vi "Cart Type Check.vi"(11 "Main References":T1) -> (1 "Cart type":string, 3 "Same Cart Type?":bool)   [LabVIEW 2020]
uses:
  Main Refs.ctl
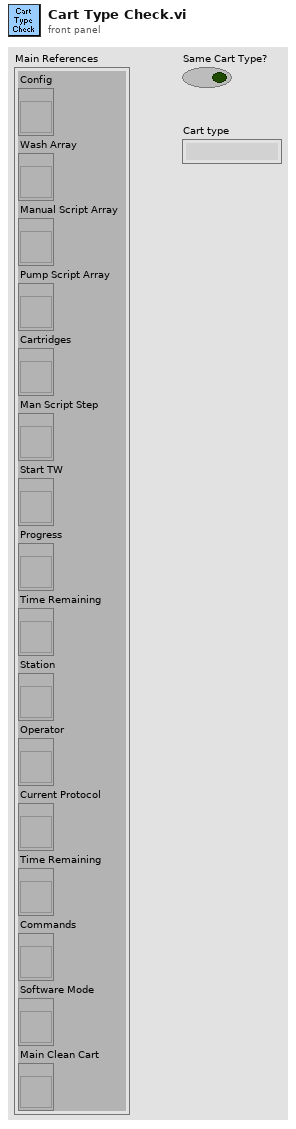
[diagram p1: front panel]
types:
  T1 = typedef "Main Refs.ctl" = cluster{"Config":refnum<vi>, "Wash Array":refnum<vi>, "Manual Script Array":refnum<vi>, "Pump Script Array":refnum<vi>, "Cartridges":refnum<vi>, "Man Script Step":refnum<vi>, "Start TW":refnum<vi>, "Progress":refnum<vi>, "Time Remaining":refnum<vi>, "Station":refnum<vi>, "Operator":refnum<vi>, "Current Protocol":refnum<vi>, "Time Remaining":refnum<vi>, "Commands":refnum<vi>, "Software Mode":refnum<vi>, "Main Clean Cart":refnum<vi>}
  T2 = typedef "Cartridges.ctl" = cluster{"Cartridge 1":T3, "Cartridge 2":T3, "Cartridge 3":T3, "Cartridge 4":T3, "Current Status":string}
  T3 = typedef "Cartridge Status.ctl" = cluster{"Serial Number":string, "Reagent":string, "Cart Status":string, "Inserted":bool, "Eject":bool}
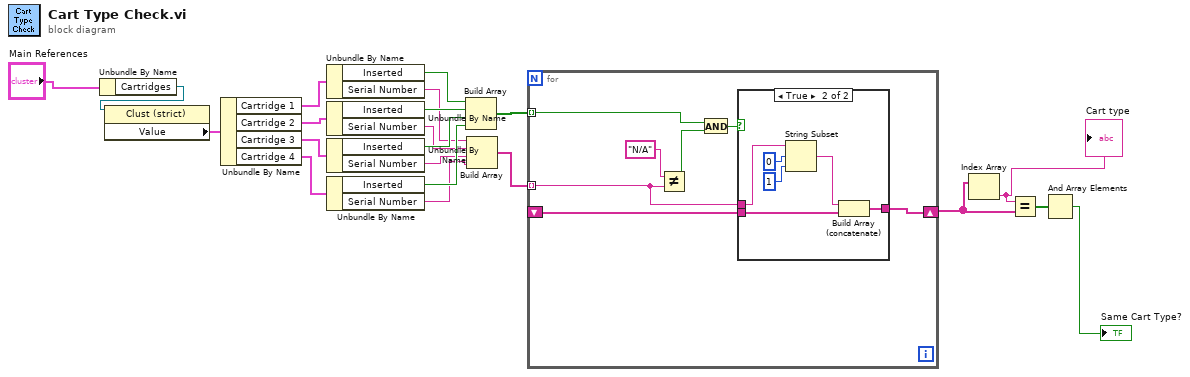
[diagram p0: block diagram]
diagram:
  n1 = Unbundle By Name("Main References") -> ("Cartridges"=w1:refnum<vi>)
  n2 = property class="Clust (strict)"(reference=w1) -> ("Value"=w21:T2)  [unwired: 1 in, 2 out]
  n3 = Unbundle By Name(w21) -> ("Cartridge 1"=w17:T3, "Cartridge 2"=w20:T3, "Cartridge 3"=w19:T3, "Cartridge 4"=w18:T3)
  n4 = Unbundle By Name(w17) -> ("Inserted"=w16:bool, "Serial Number"=w12:string)
  n5 = Unbundle By Name(w20) -> ("Inserted"=w15:bool, "Serial Number"=w11:string)
  n6 = Unbundle By Name(w19) -> ("Inserted"=w14:bool, "Serial Number"=w10:string)
  n7 = Unbundle By Name(w18) -> ("Inserted"=w13:bool, "Serial Number"=w9:string)
  n8 = Build Array(w16, w15, w14, w13) -> (w8:bool[])
  n9 = Build Array(w12, w11, w10, w9) -> (w7:string[])
  n10 = for {
    tunnel: w8 -> [w27] mode=indexing
    tunnel: w7 -> [w25] mode=indexing
    shift-right: [w24] -> w5
    shift-left: _ -> [w23]
    n11 = Not Equal?(x="N/A", y=w25) -> (x != y?=w28:bool)
    n12 = And(x=w27, y=w28) -> (x .and. y?=w26:bool)
    n13 = case shown="True" w26 {
      tunnel: w25 -> [_ w30]
      tunnel: [_ w34] -> w24
      tunnel: w23 -> [_ w33]
      frame False {
      }
      frame True {
        n14 = String Subset(string=w30, offset (0)=0, length (rest)=1 ("length (rest)")) -> (substring=w29:string)
        n15 = Build Array (concatenate)(w29, w33) -> (w34:string[])
      }
    }
  }
  n16 = Index Array(array=w5) -> (element=w3:string)  [unwired: 1 in]
  "Cart type" <- w3
  n17 = Equal?(x=w3, y=w5) -> (x = y?=w6:bool[])
  n18 = And Array Elements(Boolean array=w6) -> (logical AND=→"Same Cart Type?":bool)
